vi "Welcome.vi"() -> ()   [LabVIEW 2017]
uses:
  Globle/Login Details.vi
  Globle/Global 1.vi
  Globle/Trigger Home Screen.vi
  Globle/Login Data.vi
panel:
  in  "error in 2":errorcluster
  in  "Home":bool
  in  "Prod Analysis":bool
  in  "auto":bool
  out "error out 2":errorcluster
  in  "Remove":bool
  in  "Check":bool
  out "user name":string
  in  "Tab Control":enum32{"Page 1", "user mangement"}(tab)
  in  "LOGIN":bool
  in  "Master":bool
  in  "EXIT":bool
  in  "BD Analysis Rep":bool
  in  "USER MANGMENT":bool
  out "datetime":string
  # "Production Recording System"
  # "Designed & Developed By - NIVISION PVT LTD."
  # "Powered By-Infinity Automation Systems Pvt Ltd. Pune"
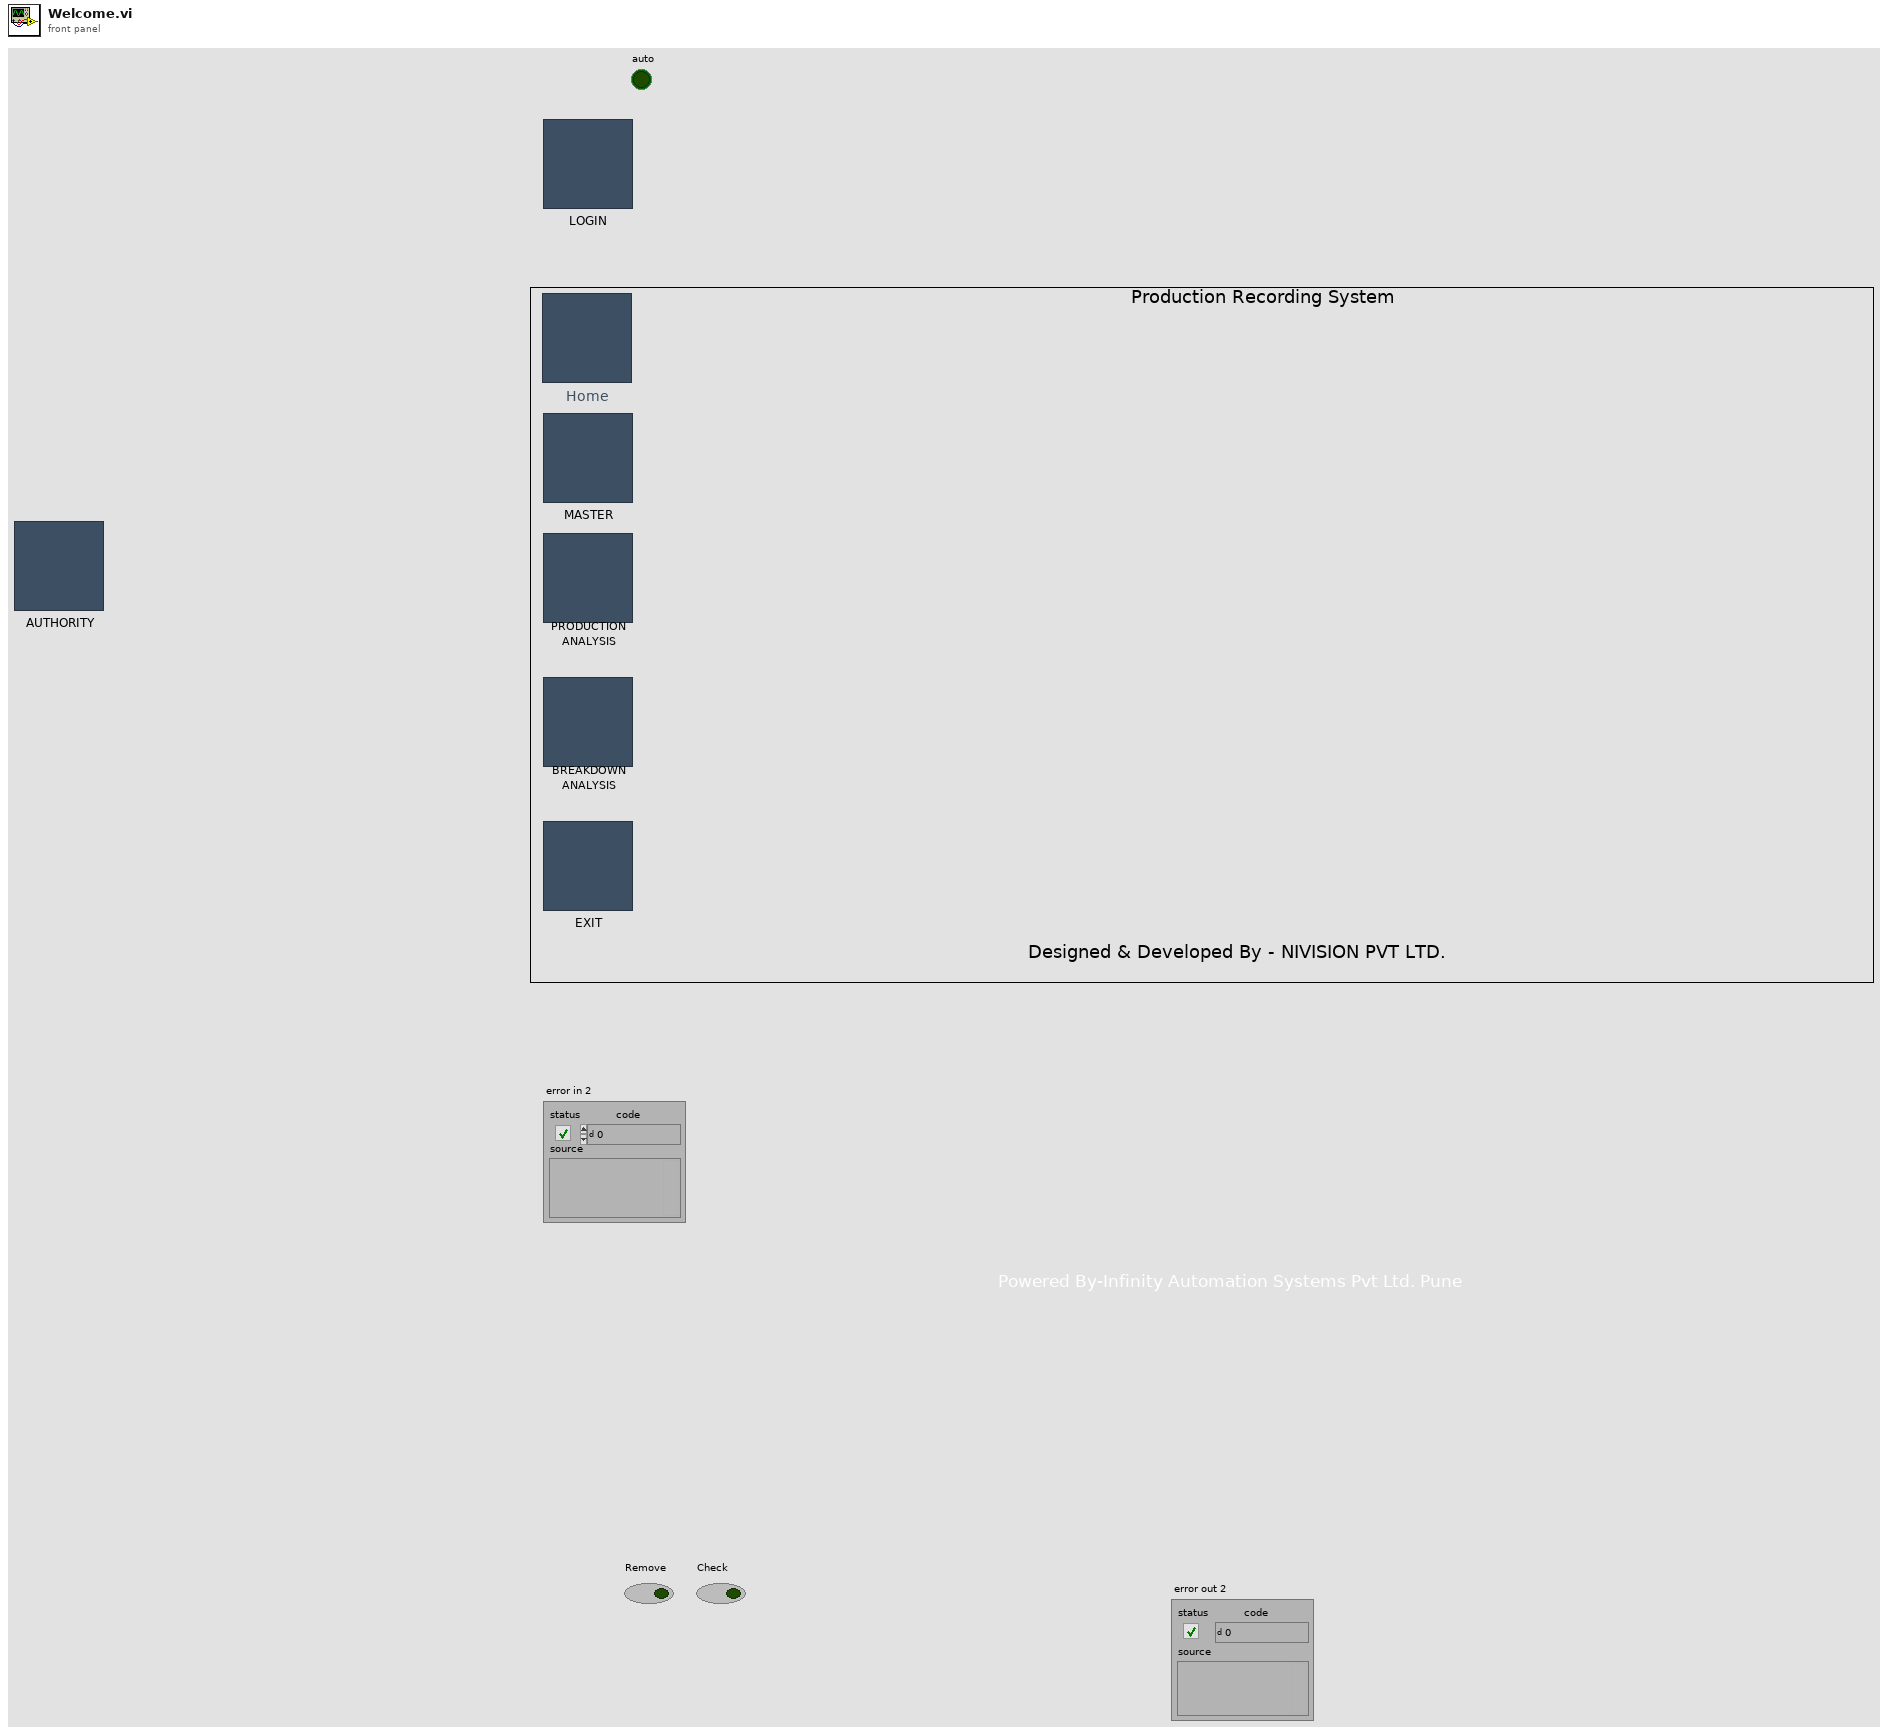
[diagram p1: front panel]
types:
  T1 = enum32{"Invalid", "Standard", "Closed", "Hidden", "Minimized", "Maximized"}
  T2 = enum8{"Enabled", "Disabled", "Disabled and Grayed Out"}
  T3 = cluster{"SCREEN 1":bool, "SCREEN 2":bool, "SCREEN 3":bool, "SCREEN 4":bool, "SCREEN 5":bool, "SCREEN 6":bool, "SCREEN 7":bool, "SCREEN 8":bool, "SCREEN 9":bool, "SCREEN 10":bool, "SCREEN 11":bool, "SCREEN 12":bool, "SCREEN 13":bool, "SCREEN 14":bool, "SCREEN 15":bool, "SCREEN 16":bool, "SCREEN 17":bool, "SCREEN 18":bool, "SCREEN 19":bool, "SCREEN 20":bool}
  T4 = enum32{"invalid app kind", "Development System", "Run Time System", "Student Edition", "Embedded LabVIEW", "Evaluation", "Custom"}
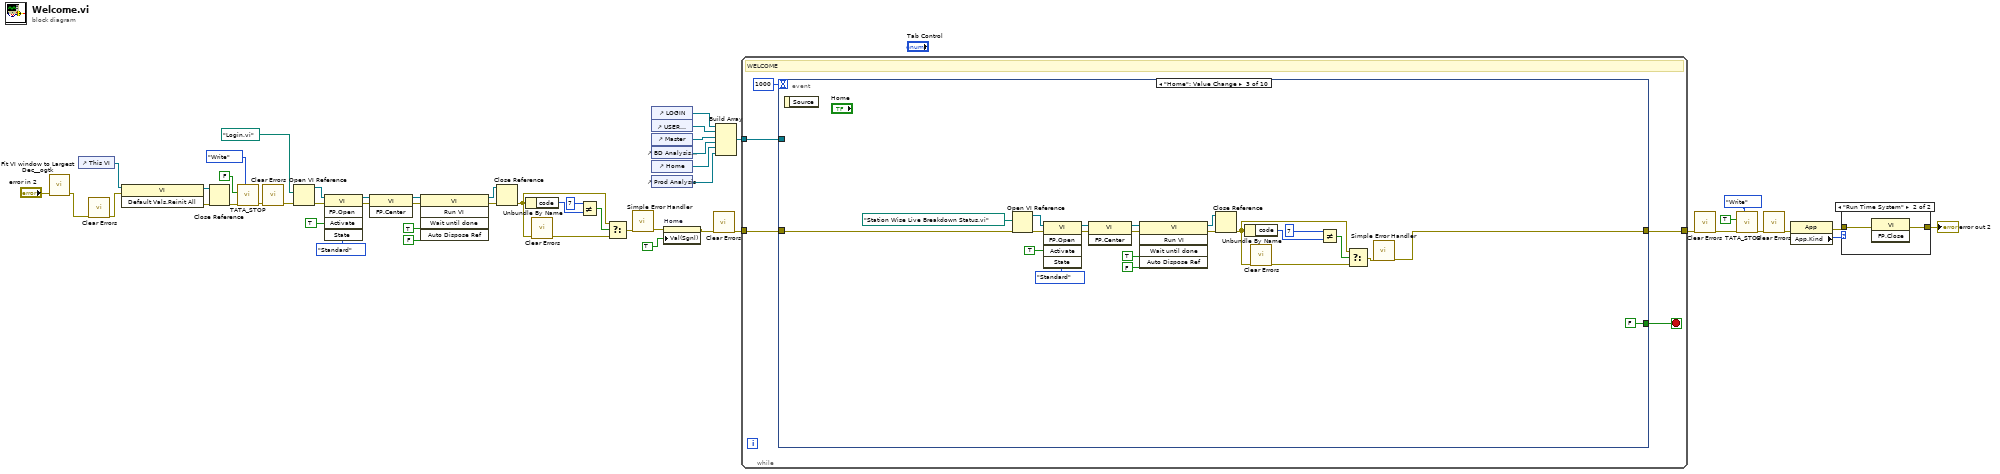
[diagram p0: block diagram]
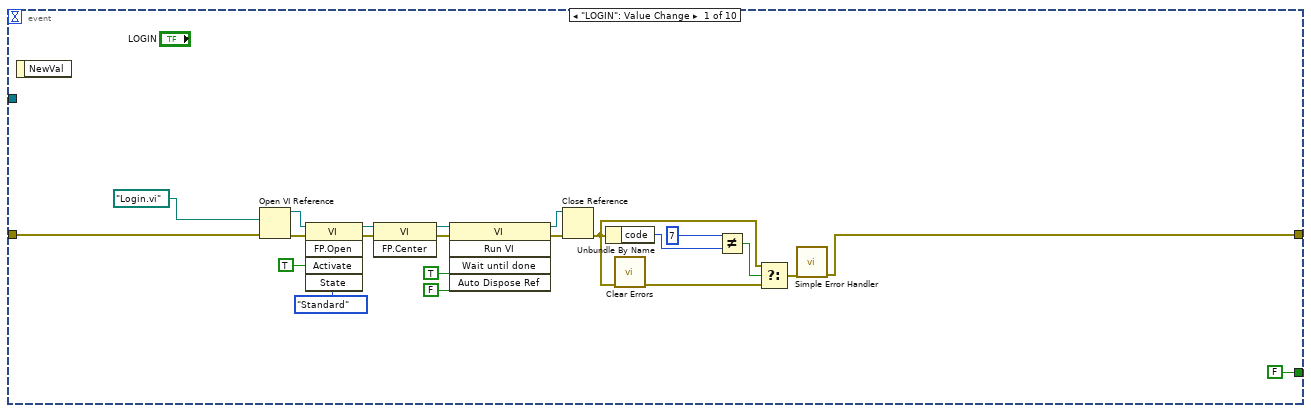
[diagram p2: hidden frame]
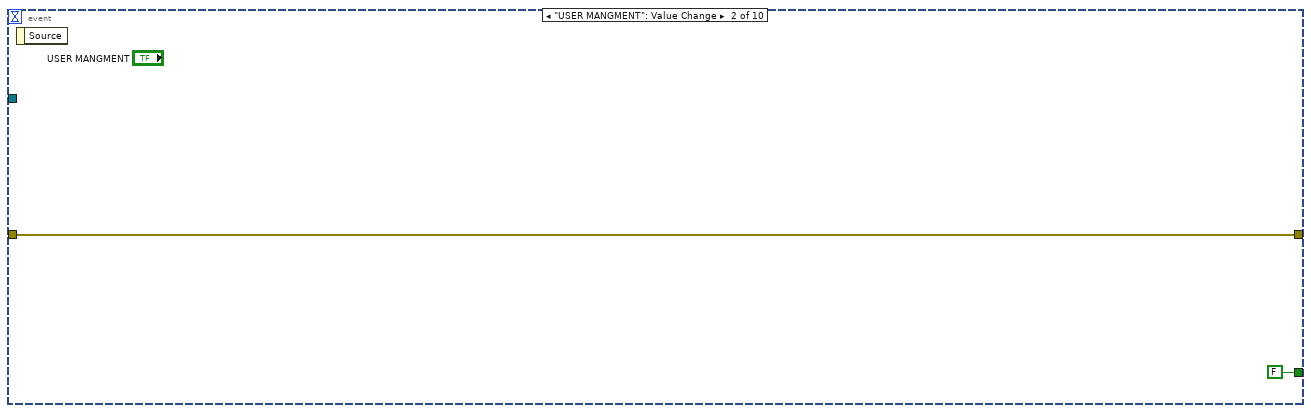
[diagram p3: hidden frame]
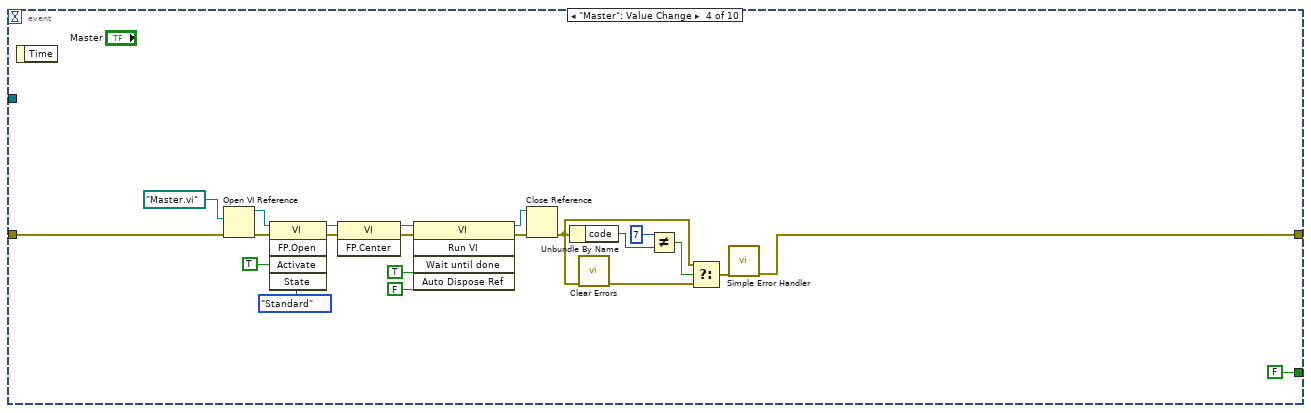
[diagram p4: hidden frame]
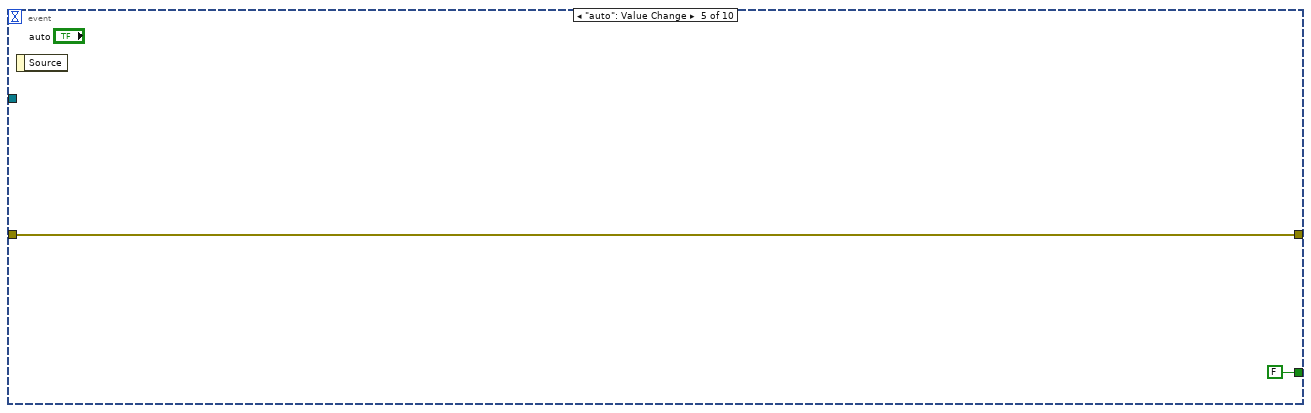
[diagram p5: hidden frame]
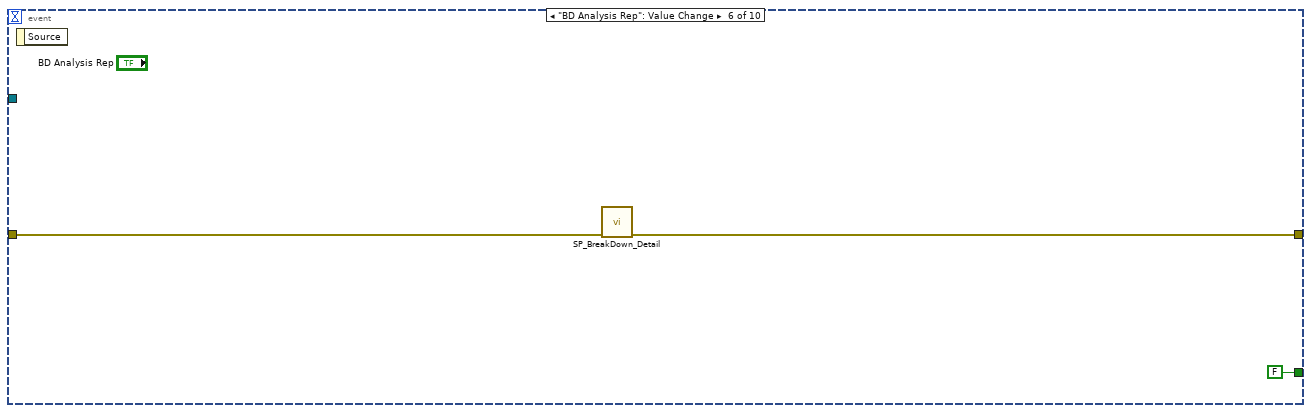
[diagram p6: hidden frame]
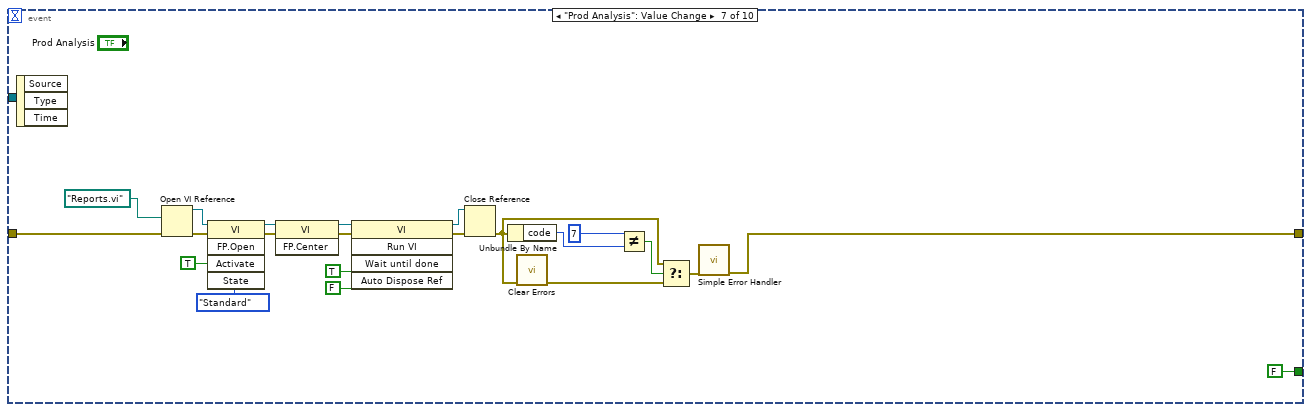
[diagram p7: hidden frame]
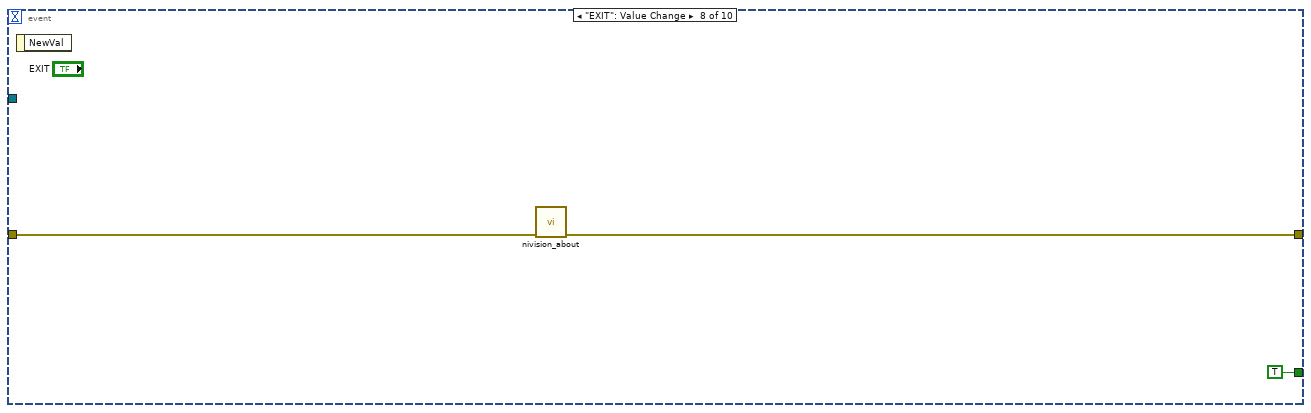
[diagram p8: hidden frame]
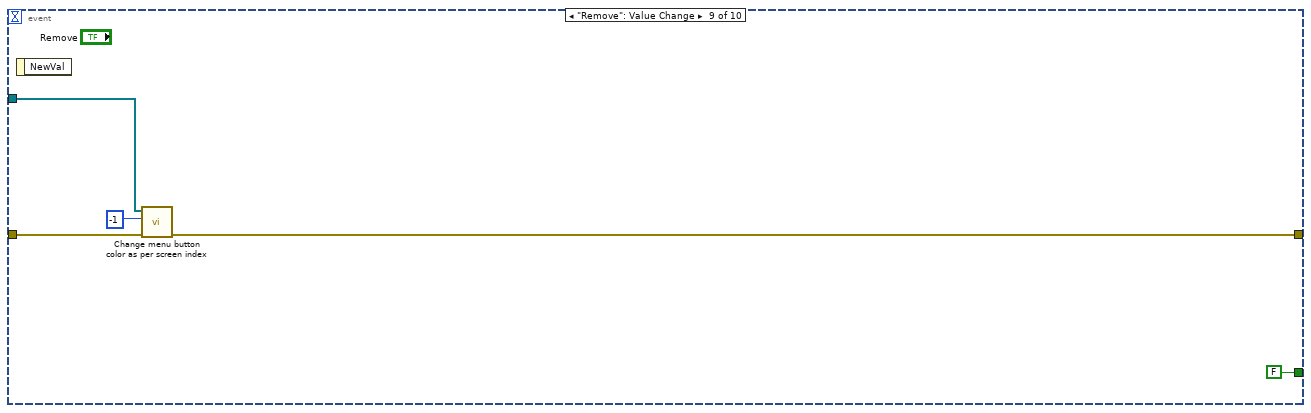
[diagram p9: hidden frame]
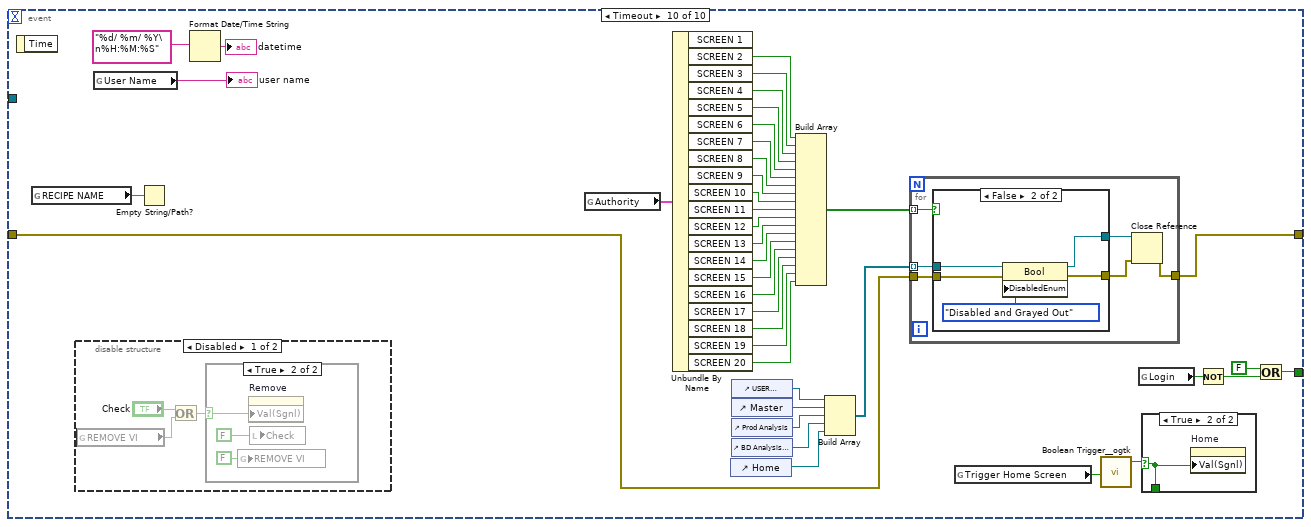
[diagram p10: hidden frame]
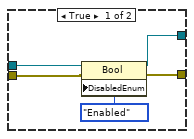
[diagram p14: hidden frame]
diagram:
  n1 = call <userlib>:"Fit VI window to Largest Dec__ogtk.vi"("error in (no error)"="error in 2") -> ("error out"=w1:errorcluster)  [unwired: 5 in, 1 out]
  n2 = control-ref of="This VI"() -> (w31:refnum<vi>)
  n3 = call <vilib>:"Clear Errors.vi"("error in (no error)"=w1) -> ("error out"=w3:errorcluster)  [unwired: 5 in, 1 out]
  n4 = invoke class="VI" method="Default Vals.Reinit All"(reference=w31, error in=w3) -> (reference out=w33:refnum<vi>, error out=w32:errorcluster)  [unwired: 1 in, 1 out]
  n5 = Close Reference(reference=w33, error in (no error)=w32) -> (error out=w34:errorcluster)
  n6 = call "TATA_STOP.vi"("Enum"=enum16{"Read", "Write"}."Write", "error in (no error)"=w34, "Boolean"=FALSE) -> ("error out"=w44:errorcluster)  [unwired: 7 in, 1 out]
  n7 = call <vilib>:"Clear Errors.vi"("error in (no error)"=w44) -> ("error out"=w7:errorcluster)  [unwired: 5 in, 1 out]
  n8 = Open VI Reference(vi path=path "Login.vi", error in (no error)=w7) -> (vi reference=w26:refnum<vi>, error out=w15:errorcluster)  [unwired: 4 in]
  n9 = invoke class="VI" method="FP.Open"(reference=w26, error in=w15, "Activate"=TRUE ("Activate?"), "State"=T1."Standard") -> (reference out=w16:refnum<vi>, error out=w21:errorcluster)  [unwired: 1 in, 3 out]
  n10 = invoke class="VI" method="FP.Center"(reference=w16, error in=w21) -> (reference out=w20:refnum<vi>, error out=w19:errorcluster)  [unwired: 1 in, 1 out]
  n11 = invoke class="VI" method="Run VI"(reference=w20, error in=w19, "Wait until done"=TRUE ("Wait Until Done"), "Auto Dispose Ref"=FALSE ("Auto Dispose Reference")) -> (reference out=w18:refnum<vi>, error out=w17:errorcluster)  [unwired: 1 in, 3 out]
  n12 = Close Reference(reference=w18, error in (no error)=w17) -> (error out=w14:errorcluster)
  n13 = Unbundle By Name(w14) -> ("code"=w22:i32)
  n14 = call <vilib>:"Clear Errors.vi"("error in (no error)"=w14) -> ("error out"=w24:errorcluster)  [unwired: 5 in, 1 out]
  n15 = Not Equal?(x=7, y=w22) -> (x != y?=w23:bool)
  n16 = Select(t=w14, s=w23, f=w24) -> (s? t:f=w25:errorcluster)
  n17 = call <vilib>:"Simple Error Handler.vi"("error in (no error)"=w25) -> ("error out"=w6:errorcluster)  [unwired: 4 in, 4 out]
  n18 = control-ref of="LOGIN"() -> (w43:refnum<vi>)
  n19 = control-ref of="USER MANGMENT"() -> (w42:refnum<vi>)
  n20 = control-ref of="Master"() -> (w37:refnum<vi>)
  n21 = control-ref of="BD Analysis Rep"() -> (w41:refnum<vi>)
  n22 = control-ref of="Home"() -> (w35:refnum<vi>)
  n23 = control-ref of="Prod Analysis"() -> (w36:refnum<vi>)
  n24 = property on="Home" class="Bool (strict)"(error in=w6, "Val(Sgnl)"=TRUE) -> (error out=w4:errorcluster)  [unwired: 1 in, 1 out]
  n25 = call <vilib>:"Clear Errors.vi"("error in (no error)"=w4) -> ("error out"=w46:errorcluster)  [unwired: 5 in, 1 out]
  n26 = Build Array(w43, w42, w37, w41, w35, w36) -> (w27:refnum<vi>[])
  n27 = while {
    tunnel: w46 -> [w51]
    tunnel: [w54] -> w45
    tunnel: w27 -> [w53]
    stop <- w52 stop-if-true
    # "WELCOME"
    n28 = event shown="[2] \"Home\": Value Change" {
      selector: _ -> [_ _ _ _ _ _ _ _ _ _]
      dyn-events: _ -> [_ _ _ _ _ _ _ _ _ _]
      timeout: 1000 -> [_ _ _ _ _ _ _ _ _ _]
      tunnel: [FALSE FALSE FALSE FALSE FALSE FALSE FALSE TRUE FALSE w159] -> w52
      tunnel: [w56 w78 w82 w103 w125 w126 w131 w151 w156 w172] -> w54
      tunnel: w53 -> [_ _ _ _ _ _ _ _ w155 _]
      tunnel: w51 -> [w57 w78 w81 w104 w125 w127 w130 w152 w154 w163]
      event "LOGIN": Value Change {
        n29 = event-data() -> ()  [unwired: 1 in, 1 out]
        n30 = Open VI Reference(vi path=path "Login.vi", error in (no error)=w57) -> (vi reference=w76:refnum<vi>, error out=w65:errorcluster)  [unwired: 4 in]
        n31 = invoke class="VI" method="FP.Open"(reference=w76, error in=w65, "Activate"=TRUE ("Activate?"), "State"=T1."Standard") -> (reference out=w66:refnum<vi>, error out=w71:errorcluster)  [unwired: 1 in, 3 out]
        n32 = invoke class="VI" method="FP.Center"(reference=w66, error in=w71) -> (reference out=w70:refnum<vi>, error out=w69:errorcluster)  [unwired: 1 in, 1 out]
        n33 = invoke class="VI" method="Run VI"(reference=w70, error in=w69, "Wait until done"=TRUE ("Wait Until Done"), "Auto Dispose Ref"=FALSE ("Auto Dispose Reference")) -> (reference out=w68:refnum<vi>, error out=w67:errorcluster)  [unwired: 1 in, 3 out]
        n34 = Close Reference(reference=w68, error in (no error)=w67) -> (error out=w64:errorcluster)
        n35 = Unbundle By Name(w64) -> ("code"=w72:i32)
        n36 = call <vilib>:"Clear Errors.vi"("error in (no error)"=w64) -> ("error out"=w74:errorcluster)  [unwired: 5 in, 1 out]
        n37 = Not Equal?(x=7, y=w72) -> (x != y?=w73:bool)
        n38 = Select(t=w64, s=w73, f=w74) -> (s? t:f=w75:errorcluster)
        n39 = call <vilib>:"Simple Error Handler.vi"("error in (no error)"=w75) -> ("error out"=w56:errorcluster)  [unwired: 4 in, 4 out]
      }
      event "USER MANGMENT": Value Change {
        n40 = event-data() -> ()  [unwired: 1 in, 1 out]
      }
      event "Home": Value Change {
        n41 = event-data() -> ()  [unwired: 1 in, 1 out]
        n42 = Open VI Reference(vi path=path "Station Wise Live Breakdown Status.vi", error in (no error)=w81) -> (vi reference=w100:refnum<vi>, error out=w89:errorcluster)  [unwired: 4 in]
        n43 = invoke class="VI" method="FP.Open"(reference=w100, error in=w89, "Activate"=TRUE ("Activate?"), "State"=T1."Standard") -> (reference out=w90:refnum<vi>, error out=w95:errorcluster)  [unwired: 1 in, 3 out]
        n44 = invoke class="VI" method="FP.Center"(reference=w90, error in=w95) -> (reference out=w94:refnum<vi>, error out=w93:errorcluster)  [unwired: 1 in, 1 out]
        n45 = invoke class="VI" method="Run VI"(reference=w94, error in=w93, "Wait until done"=TRUE ("Wait Until Done"), "Auto Dispose Ref"=FALSE ("Auto Dispose Reference")) -> (reference out=w92:refnum<vi>, error out=w91:errorcluster)  [unwired: 1 in, 3 out]
        n46 = Close Reference(reference=w92, error in (no error)=w91) -> (error out=w88:errorcluster)
        n47 = Unbundle By Name(w88) -> ("code"=w96:i32)
        n48 = call <vilib>:"Clear Errors.vi"("error in (no error)"=w88) -> ("error out"=w98:errorcluster)  [unwired: 5 in, 1 out]
        n49 = Not Equal?(x=7, y=w96) -> (x != y?=w97:bool)
        n50 = Select(t=w88, s=w97, f=w98) -> (s? t:f=w99:errorcluster)
        n51 = call <vilib>:"Simple Error Handler.vi"("error in (no error)"=w99) -> ("error out"=w82:errorcluster)  [unwired: 4 in, 4 out]
      }
      event "Master": Value Change {
        n52 = event-data() -> ()  [unwired: 1 in, 1 out]
        n53 = Open VI Reference(vi path=path "Master.vi", error in (no error)=w104) -> (vi reference=w122:refnum<vi>, error out=w111:errorcluster)  [unwired: 4 in]
        n54 = invoke class="VI" method="FP.Open"(reference=w122, error in=w111, "Activate"=TRUE ("Activate?"), "State"=T1."Standard") -> (reference out=w112:refnum<vi>, error out=w117:errorcluster)  [unwired: 1 in, 3 out]
        n55 = invoke class="VI" method="FP.Center"(reference=w112, error in=w117) -> (reference out=w116:refnum<vi>, error out=w115:errorcluster)  [unwired: 1 in, 1 out]
        n56 = invoke class="VI" method="Run VI"(reference=w116, error in=w115, "Wait until done"=TRUE ("Wait Until Done"), "Auto Dispose Ref"=FALSE ("Auto Dispose Reference")) -> (reference out=w114:refnum<vi>, error out=w113:errorcluster)  [unwired: 1 in, 3 out]
        n57 = Close Reference(reference=w114, error in (no error)=w113) -> (error out=w110:errorcluster)
        n58 = Unbundle By Name(w110) -> ("code"=w118:i32)
        n59 = call <vilib>:"Clear Errors.vi"("error in (no error)"=w110) -> ("error out"=w120:errorcluster)  [unwired: 5 in, 1 out]
        n60 = Not Equal?(x=7, y=w118) -> (x != y?=w119:bool)
        n61 = Select(t=w110, s=w119, f=w120) -> (s? t:f=w121:errorcluster)
        n62 = call <vilib>:"Simple Error Handler.vi"("error in (no error)"=w121) -> ("error out"=w103:errorcluster)  [unwired: 4 in, 4 out]
      }
      event "auto": Value Change {
        n63 = event-data() -> ()  [unwired: 1 in, 1 out]
      }
      event "BD Analysis Rep": Value Change {
        n64 = event-data() -> ()  [unwired: 1 in, 1 out]
        n65 = call "SP_BreakDown_Detail.vi"("error in (no error)"=w127) -> ("error out"=w126:errorcluster)  [unwired: 10 in]
      }
      event "Prod Analysis": Value Change {
        n66 = event-data() -> ()  [unwired: 1 in, 3 out]
        n67 = Open VI Reference(vi path=path "Reports.vi", error in (no error)=w130) -> (vi reference=w149:refnum<vi>, error out=w138:errorcluster)  [unwired: 4 in]
        n68 = invoke class="VI" method="FP.Open"(reference=w149, error in=w138, "Activate"=TRUE ("Activate?"), "State"=T1."Standard") -> (reference out=w139:refnum<vi>, error out=w144:errorcluster)  [unwired: 1 in, 3 out]
        n69 = invoke class="VI" method="FP.Center"(reference=w139, error in=w144) -> (reference out=w143:refnum<vi>, error out=w142:errorcluster)  [unwired: 1 in, 1 out]
        n70 = invoke class="VI" method="Run VI"(reference=w143, error in=w142, "Wait until done"=TRUE ("Wait Until Done"), "Auto Dispose Ref"=FALSE ("Auto Dispose Reference")) -> (reference out=w141:refnum<vi>, error out=w140:errorcluster)  [unwired: 1 in, 3 out]
        n71 = Close Reference(reference=w141, error in (no error)=w140) -> (error out=w137:errorcluster)
        n72 = Unbundle By Name(w137) -> ("code"=w145:i32)
        n73 = call <vilib>:"Clear Errors.vi"("error in (no error)"=w137) -> ("error out"=w147:errorcluster)  [unwired: 5 in, 1 out]
        n74 = Not Equal?(x=7, y=w145) -> (x != y?=w146:bool)
        n75 = Select(t=w137, s=w146, f=w147) -> (s? t:f=w148:errorcluster)
        n76 = call <vilib>:"Simple Error Handler.vi"("error in (no error)"=w148) -> ("error out"=w131:errorcluster)  [unwired: 4 in, 4 out]
      }
      event "EXIT": Value Change {
        n77 = event-data() -> ()  [unwired: 1 in, 1 out]
        n78 = call "nivision_about.vi"("error in (no error)"=w152) -> ("error out"=w151:errorcluster)  [unwired: 10 in]
      }
      event "Remove": Value Change {
        n79 = event-data() -> ()  [unwired: 1 in, 1 out]
        n80 = call "Change menu button color as per screen index.vi"("error in (no error)"=w154, "Screen Index"=-1, "Array"=w155) -> ("error out"=w156:errorcluster)  [unwired: 8 in]
      }
      event Timeout {
        n81 = event-data() -> ()  [unwired: 1 in, 1 out]
        n82 = global read "Global 1.vi" "RECIPE NAME"() -> (w174:string)
        n83 = disable-structure shown="Disabled" {
          frame Disabled {
            n84 = global read "Global 1.vi" "REMOVE VI"() -> (w200:bool)
            n85 = Or(x="Check", y=w200) -> (x .or. y?=w201:bool)
            n86 = case shown="True" w201 {
              selector: w201 -> [_ w205]
              frame False {
              }
              frame True {
                n87 = global write "Global 1.vi" "REMOVE VI"(FALSE ("remove_VI")) -> ()
                n88 = property on="Remove" class="Bool (strict)"("Val(Sgnl)"=w205) -> ()  [unwired: 2 in, 2 out]
                n89 = local write "Check"(FALSE ("Check")) -> ()
              }
            }
          }
          frame Enabled {
          }
        }
        n90 = global read "Login Details.vi" "User Name"() -> (→"user name":string)
        n91 = Empty String/Path?(string/path=w174) -> ()  [unwired: 1 out]
        n92 = Format Date/Time String(time format string (%c)="%d/ %m/ %Y\n%H:%M:%S") -> (date/time string=→"datetime":string)  [unwired: 2 in]
        n93 = global read "Login Details.vi" "Authority"() -> (w171:T3)
        n94 = Unbundle By Name(w171) -> ("SCREEN 2"=w193:bool, "SCREEN 3"=w192:bool, "SCREEN 4"=w191:bool, "SCREEN 5"=w190:bool, "SCREEN 6"=w189:bool, "SCREEN 7"=w188:bool, "SCREEN 8"=w187:bool, "SCREEN 9"=w186:bool, "SCREEN 10"=w185:bool, "SCREEN 11"=w184:bool, "SCREEN 12"=w183:bool, "SCREEN 13"=w182:bool, "SCREEN 14"=w181:bool, "SCREEN 15"=w180:bool, "SCREEN 16"=w179:bool, "SCREEN 17"=w178:bool, "SCREEN 18"=w177:bool, "SCREEN 19"=w176:bool, "SCREEN 20"=w175:bool)  [unwired: 1 out]
        n95 = control-ref of="Home"() -> (w164:refnum<vi>)
        n96 = control-ref of="USER MANGMENT"() -> (w168:refnum<vi>)
        n97 = control-ref of="Master"() -> (w169:refnum<vi>)
        n98 = control-ref of="Prod Analysis"() -> (w167:refnum<vi>)
        n99 = control-ref of="BD Analysis Rep"() -> (w170:refnum<vi>)
        n100 = Build Array(w193, w192, w191, w190, w189, w188, w187, w186, w185, w184, w183, w182, w181, w180, w179, w178, w177, w176, w175) -> (w194:bool[])
        n101 = Build Array(w168, w169, w167, w170, w164) -> (w173:refnum<vi>[])
        n102 = for {
          tunnel: w194 -> [w206] mode=indexing
          tunnel: w173 -> [w211] mode=indexing
          tunnel: w163 -> [w210]
          tunnel: [w208] -> w172
          n103 = case shown="False" w206 {
            tunnel: w211 -> [w215 w220]
            tunnel: w210 -> [w214 w219]
            tunnel: [w213 w218] -> w209
            tunnel: [w212 w217] -> w207
            frame True {
              n104 = property class="Bool"(reference=w215, error in=w214, "DisabledEnum"=T2."Enabled" ("Disabled")) -> (reference out=w212:refnum<vi>, error out=w213:errorcluster)
            }
            frame False {
              n105 = property class="Bool"(reference=w220, error in=w219, "DisabledEnum"=T2."Disabled and Grayed Out" ("Disabled")) -> (reference out=w217:refnum<vi>, error out=w218:errorcluster)
            }
          }
          n106 = Close Reference(reference=w207, error in (no error)=w209) -> (error out=w208:errorcluster)
        }
        n107 = global read "Trigger Home Screen.vi" "Trigger Home Screen"() -> (w166:bool)
        n108 = call <userlib>:"Boolean Trigger__ogtk.vi"("Boolean Input"=w166) -> ("Rising Edge"=w165:bool)  [unwired: 1 in, 1 out]
        n109 = global read "Login Data.vi" "Login"() -> (w162:bool)
        n110 = case shown="True" w165 {
          selector: w165 -> [w198 w199]
          tunnel: [w198 w199] -> _
          frame False {
          }
          frame True {
            n111 = property on="Home" class="Bool (strict)"("Val(Sgnl)"=w199) -> ()  [unwired: 2 in, 2 out]
          }
        }
        n112 = Not(x=w162) -> (.not. x?=w161:bool)
        n113 = Or(x=FALSE, y=w161) -> (x .or. y?=w159:bool)
      }
    }
  }
  n114 = call <vilib>:"Clear Errors.vi"("error in (no error)"=w45) -> ("error out"=w28:errorcluster)  [unwired: 5 in, 1 out]
  n115 = call "TATA_STOP.vi"("Enum"=enum16{"Read", "Write"}."Write", "error in (no error)"=w28, "Boolean"=TRUE) -> ("error out"=w38:errorcluster)  [unwired: 7 in, 1 out]
  n116 = call <vilib>:"Clear Errors.vi"("error in (no error)"=w38) -> ("error out"=w48:errorcluster)  [unwired: 5 in, 1 out]
  n117 = property class="App"(error in=w48) -> (error out=w49:errorcluster, "App.Kind"=w50:T4)  [unwired: 1 in, 1 out]
  n118 = case shown="\"Run Time System\"" w50 {
    tunnel: w49 -> [w222 w224]
    tunnel: [w222 w223] -> w47
    frame Default {
    }
    frame "Run Time System" {
      n119 = invoke class="VI" method="FP.Close"(error in=w224) -> (error out=w223:errorcluster)  [unwired: 2 in, 2 out]
    }
  }
  "error out 2" <- w47
